vi "Set Report Tab Width.vi"(0 "report in":refnum<class "NI_Standard Report.lvclass">, 5 "width (.25)":dbl=0.25 format="%.2f", 9 "measurement system (US)":u16(ring)=1 items=["US", "Metric"], 11 "error in (no error)":errorcluster) -> (4 "report out":refnum<class "NI_Standard Report.lvclass">, 15 "error out":errorcluster)   [LabVIEW 2020, in "NI_Standard Report.lvclass"]
doc: "LabVIEW no longer supports this VI.\n\nSets the tab width in the report. You cannot use this VI with HTML reports.\n\nTo place a tab in the text, insert the token <tab> in the text string. Alternatively, you can use the Concatenate Strings function and insert a tab constant to build the text string."
uses:
  <vilib>/Utility/NIReport.llb/Standard Report/NI_Standard Report.lvclass
panel:
  in  "warning msg":string="Setting the tab width of a Standard Report is no longer supported."
  # "LabVIEW no longer supports this VI."
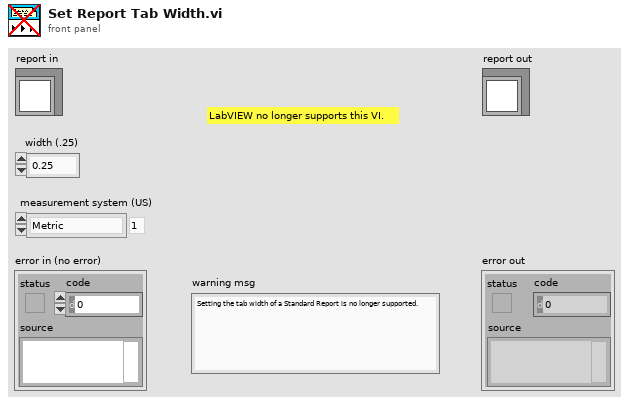
[diagram p1: front panel]
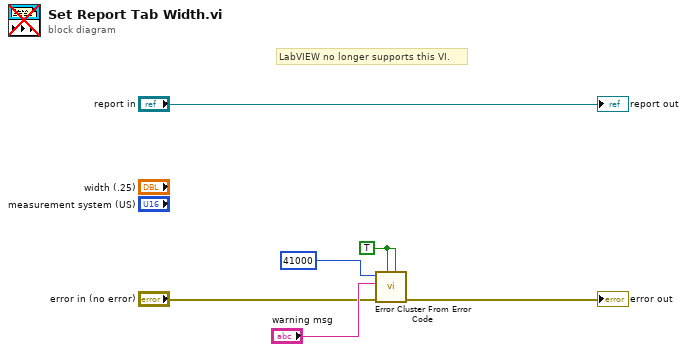
[diagram p0: block diagram]
diagram:
  w4 = TRUE ("is warning? (False)")
  # "LabVIEW no longer supports this VI."
  n1 = call <vilib>:"Error Cluster From Error Code.vi"("is warning? (False)"=w4, "show call chain? (False)"=w4, "error in (no error)"="error in (no error)", "error message (\"\")"="warning msg", "error code (0)"=41000) -> ("error out"=→"error out":errorcluster)  [unwired: 4 in]
  "report out" <- "report in"
